vi "Set Number of Test Runners.vi"(8 "error in (no error)":errorcluster, 10 "Number of Test Runners":u32=1, 11 "Test Runner in":refnum<class "Test Runner.lvclass">) -> (0 "error out":errorcluster, 3 "Test Runner out":refnum<class "Test Runner.lvclass">)   [LabVIEW 2020, in "Test Runner.lvclass"]
uses:
  Test Runner.lvclass
  C:/Git/astemes-lunit/source/Application Framework/Process Classes/Process/Process.lvclass
  Application Framework/Process Classes/Process/Process.lvclass/Process.ctl
  Application Framework/Process Classes/Process/Process.lvclass
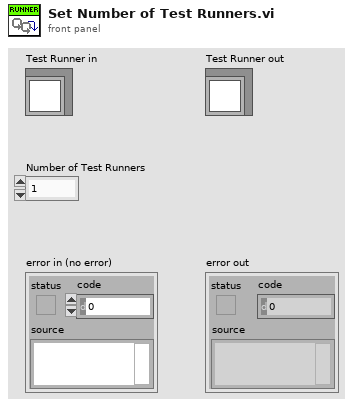
[diagram p1: front panel]
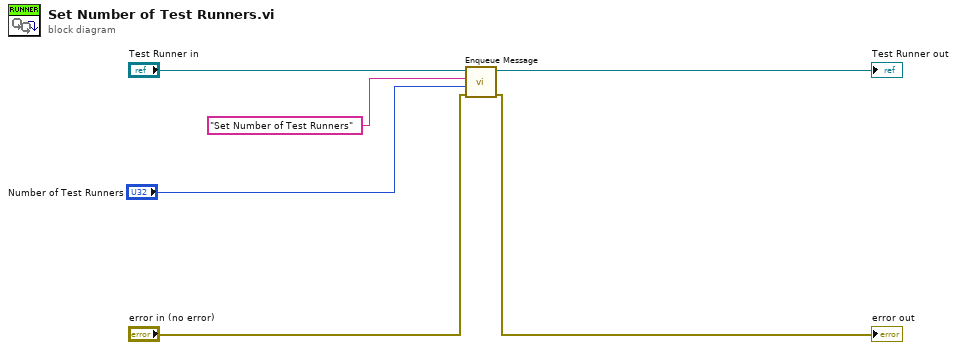
[diagram p0: block diagram]
diagram:
  n1 = call "Enqueue Message.vi"("error in (no error)"="error in (no error)", "Message Data"="Number of Test Runners", "Message"="Set Number of Test Runners", "Process In"="Test Runner in") -> ("error out"=→"error out":errorcluster, "Process Out"=→"Test Runner out":refnum<class "Test Runner.lvclass">)  [unwired: 6 in]
